vi "DAQmx Create Strain Rosette AI Channels (sub).vi"(0 "task in":refnum<k21>, 1 "virtual channel name":string, 5 "physical channel name":tag, 7 "rosette type":i32(ring)=15968 items=["Rectangular Rosette"=15968, "Delta Rosette"=15969, "Tee Rosette"=15970], 9 "rosette measurements":i32[](array[ring]) items=["Principal Strain 1"=15971, "Principal Strain 2"=15972, "Principal Strain Angle"=15973, "Cartesian Strain X"=15974, "Cartesian Strain Y"=15975, "Cartesian Shear Strain XY"=15976, "Maximum Shear Strain"=15977, "Maximum Shear Strain Angle"=15978], 11 "error in":errorcluster, 12 "gage orientation":dbl) -> (4 "task out":refnum<k21>, 6 "raw strain channels":string, 8 "calculated strain channels":string, 15 "error out":errorcluster)   [LabVIEW 2013]
uses:
  nilvaiu.dll
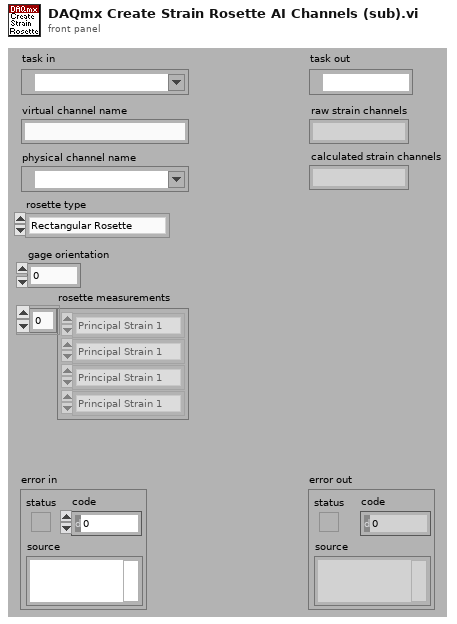
[diagram p1: front panel]
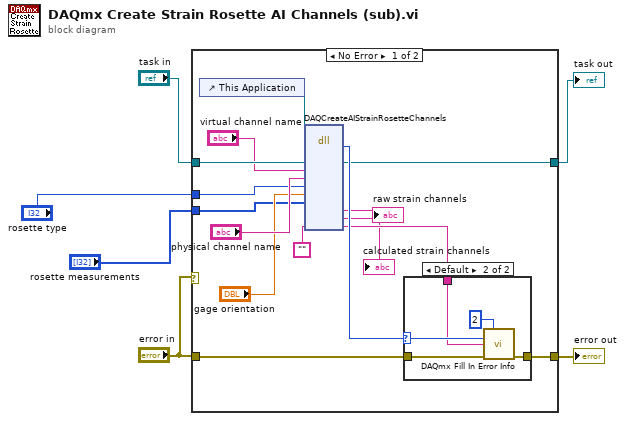
[diagram p0: block diagram]
diagram:
  n1 = case shown="No Error" "error in" {
    tunnel: [w19 w29] -> w6
    tunnel: "error in" -> [w21 w29]
    tunnel: "task in" -> [w17 w28]
    tunnel: [w11 w28] -> w3
    tunnel: "rosette type" -> [w9 _]
    tunnel: "rosette measurements" -> [w7 _]
    frame No Error {
      n2 = control-ref of="This Application"() -> (w12:refnum<vi>)
      n3 = dll-call lib="nilvaiu.*" fn="DAQCreateAIStrainRosetteChannels"("lvAppReference"=w12, "taskID"=w17, "virtual channel name"="virtual channel name", "physical channel name"="physical channel name", "rosetteType"=w9, "gageOrientation"="gage orientation", "rosetteMeasurements"=w7, "extendedErrorIndo"="") -> ("return type"=w20:i32, "taskID"=w11:refnum<k21>, "rawChannelNamesOut"=→"raw strain channels":string, "calculatedChannelNamesOut"=→"calculated strain channels":string, "extendedErrorIndo"=w13:string)  [unwired: 9 in, 4 out]
      n4 = case shown="Default" w20 {
        selector: w20 -> [_ w25]
        tunnel: w21 -> [w22 w27]
        tunnel: [w22 w26] -> w19
        tunnel: w13 -> [_ w23]
        frame 0 {
        }
        frame Default {
          n5 = call "DAQmx Fill In Error Info.vi"("depth"=2, "status code"=w25, "extended error info"=w23, "error in"=w27) -> ("error out"=w26:errorcluster)  [unwired: 1 in, 10 out]
        }
      }
    }
    frame Error {
    }
  }
  "error out" <- w6
  "task out" <- w3
